vi "LVClass_HasoSlopes equalize AB.vi"(0 "HasoSlopes dest in":refnum<class "HasoSlopes.lvclass">, 5 "HasoSlopes source in":refnum<class "HasoSlopes.lvclass">, 11 "error in (no error)":errorcluster) -> (4 "HasoSlopes dest out":refnum<class "HasoSlopes.lvclass">, 6 "HasoSlopes source out":refnum<class "HasoSlopes.lvclass">, 15 "error out":errorcluster)   [LabVIEW 2020, in "HasoSlopes.lvclass"]
doc: "HasoSlopes assignment.\n\n--------------------------------------------------------------------------------\n\n<B>HasoSlopes_dstIn </B> : HasoSlopes object to assign.\n<B>HasoSlopes_dstOut </B> : HasoSlopes object to assign.\n<B>HasoSlopes_src </B> : HasoSlopes object to copy.\n<B>ErrorIn </B> : Error\n<B>ErrorOut </B> : Error\n\n--------------------------------------------------------------------------------"
uses:
  HasoSlopes.lvclass
  HasoSlopes.lvclass/HasoSlopes.ctl
  LVClass_HasoSlopes Read HasoSlopes _ property.vi
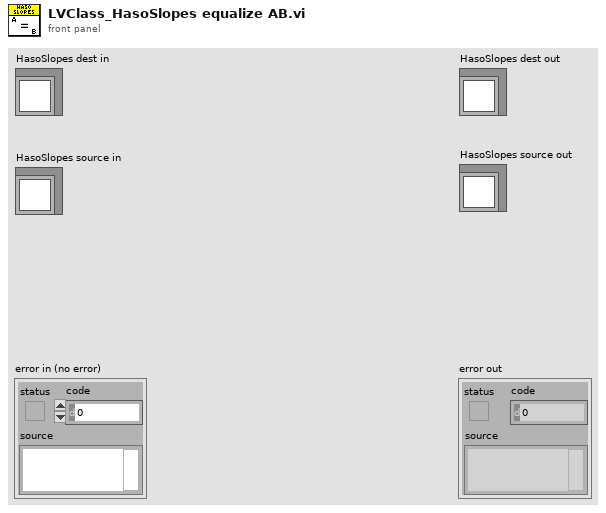
[diagram p1: front panel]
types:
  T1 = typedef "ClassID.ctl" = i64
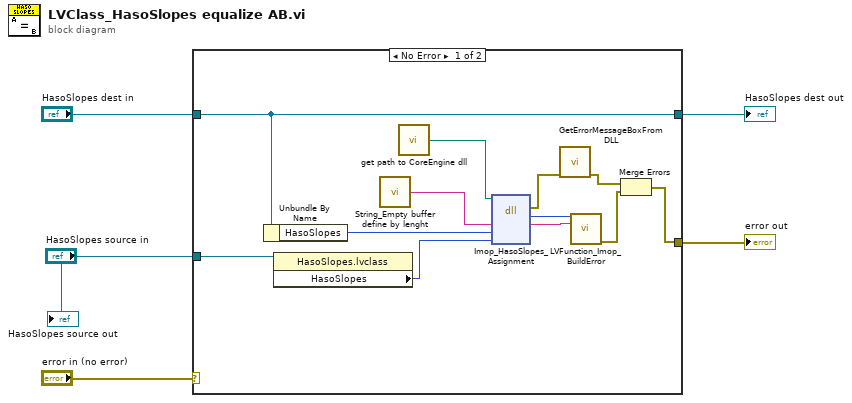
[diagram p0: block diagram]
diagram:
  n1 = case shown="No Error" "error in (no error)" {
    selector: "error in (no error)" -> [_ w19]
    tunnel: [w6 w19] -> w5
    tunnel: [w11 w18] -> w4
    tunnel: "HasoSlopes dest in" -> [w11 w18]
    tunnel: "HasoSlopes source in" -> [w10 _]
    frame No Error {
      n2 = Unbundle By Name(w11) -> ("HasoSlopes"=w12:T1)
      n3 = property class="HasoSlopes.lvclass"(reference=w10) -> ("HasoSlopes"=w9:T1)  [unwired: 1 in, 2 out]
      n4 = call "String_Empty buffer define by lenght.vi"() -> ("Empty buffer"=w17:string)  [unwired: 1 in]
      n5 = call "get path to CoreEngine dll.vi"() -> ("path to wavekit library"=w14:path)  [unwired: 14 in, 1 out]
      n6 = dll-call lib="D:/soft/HASO_v3/SVN_trunk/ImOpCoreEngine4_LV2011/DLLs/c_interface_vc100.dll" fn="Imop_HasoSlopes_Assignment"(path in=w14, "message"=w17, "objet"=w12, "hasoslopesb"=w9) -> (error out=w13:errorcluster, "return type"=w15:i32, "message"=w16:string)  [unwired: 4 in, 1 out]
      n7 = call "GetErrorMessageBoxFromDLL.vi"("error IN"=w13) -> ("error OUT"=w8:errorcluster)  [unwired: 10 in]
      n8 = call "LVFunction_Imop_BuildError.vi"("code"=w15, "String to Prepend to source (\"\")"=w16) -> ("error out"=w7:errorcluster)  [unwired: 13 in]
      n9 = Merge Errors(w8, w7) -> (w6:errorcluster)
    }
    frame Error {
    }
  }
  "error out" <- w5
  "HasoSlopes dest out" <- w4
  "HasoSlopes source out" <- "HasoSlopes source in"
